vi "Fan Acceleration Curve J&J.vi"() -> ()   [LabVIEW 2015]
uses:
  <vilib>/Platform/TimedLoop/XDataNode/timing_clust.ctl
  <vilib>/Platform/TimedLoop/XDataNode/nitl_modes.ctl
  <vilib>/Platform/TimedLoop/XDataNode/wakeup.ctl
  <vilib>/platform/TimedLoop/XDataNode/XDataNode.xnode
  <vilib>/Platform/TimedLoop/XDataNode/XDNodeRunTimeDep.lvlib
panel:
  out "Countrate":cluster{i32[], i32[]}(graph)
  in  "Controls":T1
  in  "stop":bool
  out "counts per Time Increment":dbl(knob) scale=0.0..100.0
  out "output cluster":cluster{i32, dbl}
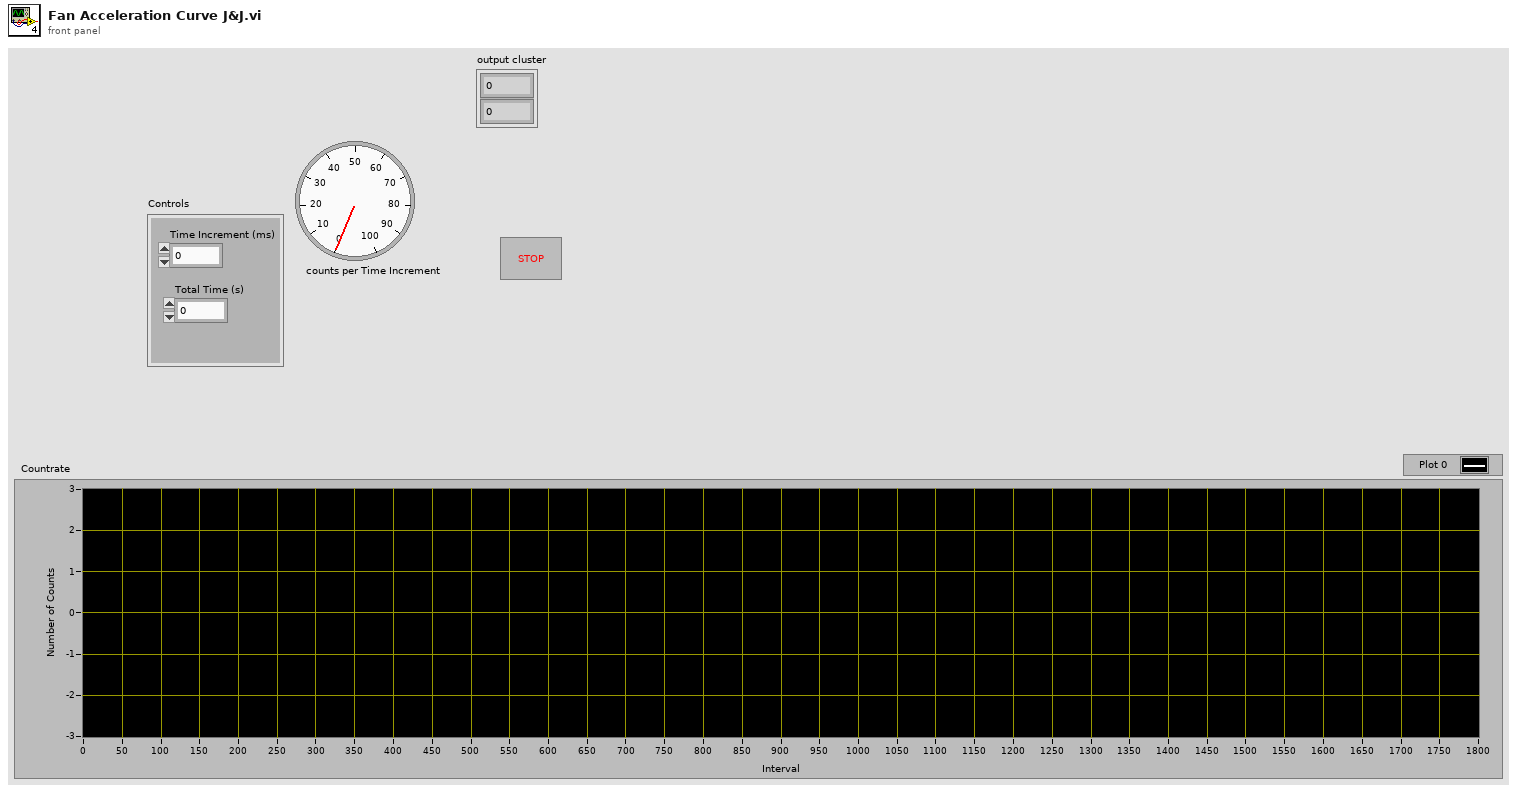
[diagram p1: front panel]
types:
  T1 = cluster{"Time Increment (ms)":i64, "Total Time (s)":dbl}
  T2 = enum16{"open", "replace", "create", "open or create", "replace or create", "replace or create with confirmation"}
  T3 = typedef "XDNodeRunTimeDep.lvlib/timing_clust.ctl" = cluster{"Expected End [f-1]":u64, "Actual End [f-1]":u64, "Finished Late? [f-1]":bool, "Expected End [i-1]":u64, "Actual End [i-1]":u64, "Finished Late? [i-1]":bool, "Expected Start [i]":u64, "Actual Start [i]":u64, "Expected Start [f]":u64, "Actual Start [f]":u64, "Source Name":string, "Structure Name":string, "Period":i64, "Deadline":i64, "Offset":i64, "Start":i64, "Priority":i32, "Timeout":i32, "Mode":T4, "Wakeup Reason":T5, "Error":errorcluster, "Source Type":string, "Secondary Source Type":string, "Global End Time":u64, "Global Start Time":u64, "Frame Duration":u64, "Iteration Duration":u64, "Assigned CPU":i32, "I/O Scan Engine Mode":u32}
  T4 = typedef "XDNodeRunTimeDep.lvlib/nitl_modes.ctl" = enum32{"No Change", "Process missed periods, maintain original phase", "Discard missed periods, maintain original phase", "Process missed periods, ignore original phase", "Discard missed periods, ignore original phase"}
  T5 = typedef "XDNodeRunTimeDep.lvlib/wakeup.ctl" = enum32{"Normal", "Aborted", "Asynchronous wakeup", "Timing source error", "Timed loop error", "Timeout"}
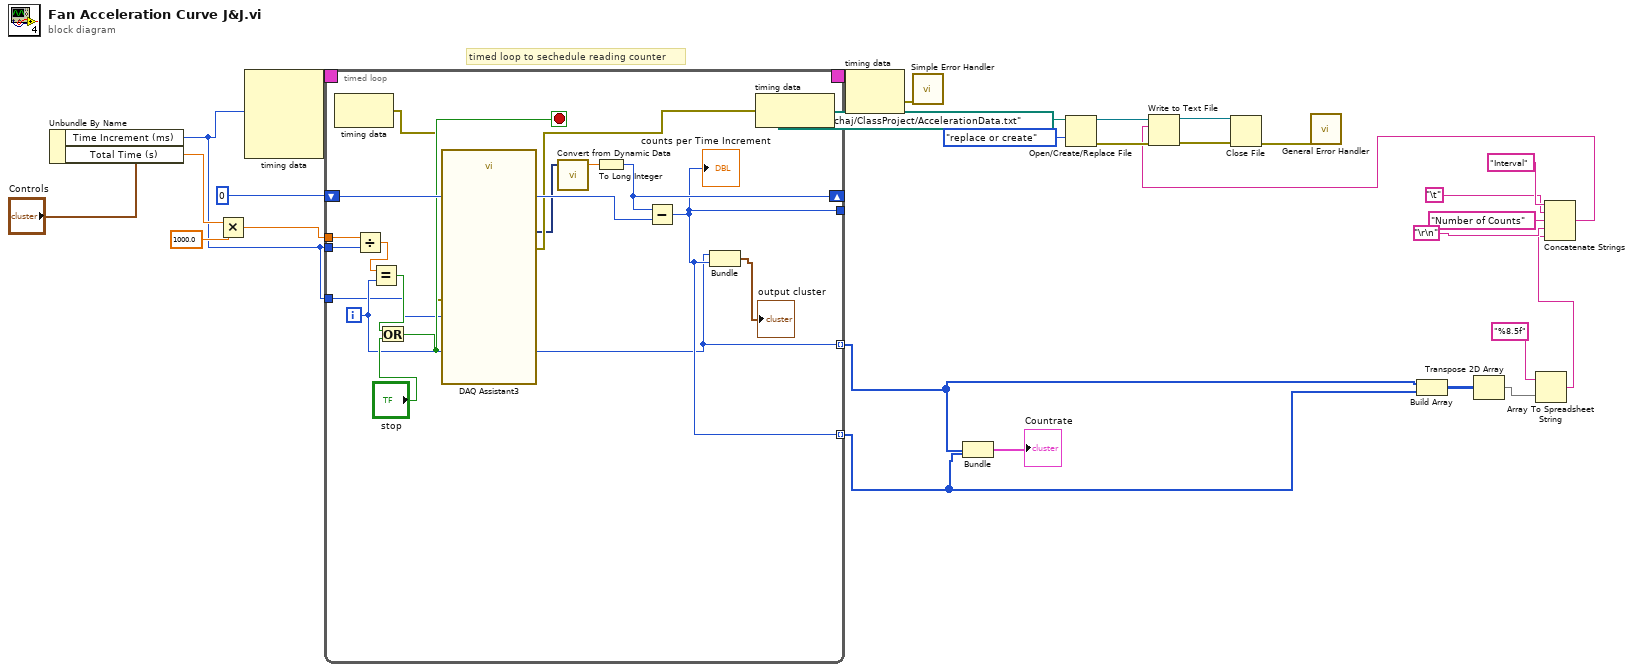
[diagram p0: block diagram]
diagram:
  # "timed loop to sechedule reading counter"
  n1 = Unbundle By Name("Controls") -> ("Time Increment (ms)"=w1:i64, "Total Time (s)"=w23:dbl)
  n2 = Multiply(x=w23, y=1000.0) -> (x*y=w21:dbl)
  n3 = node-c288(w1) -> (w28:T3)  [unwired: 3 in]
  n4 = timed-loop {
    timing: w28 -> [_]
    timing-out: [_] -> w27
    shift-right: [w44] -> _
    shift-left: 0 -> [w36]
    tunnel: [w38] -> _
    tunnel: w1 -> [w30]
    tunnel: w21 -> [w42]
    tunnel: [w38] -> w2 mode=indexing
    tunnel: [w37] -> w3 mode=indexing
    tunnel: w1 -> [w29]
    i -> [w37]
    stop <- w35 stop-if-true
    n5 = node-c288() -> (w33:errorcluster)  [unwired: 1 in]
    n6 = Divide(x=w42, y=w30) -> (x/y=w34:dbl)
    n7 = Equal?(x=w34, y=w37) -> (x = y?=w40:bool)
    n8 = Or(x=w40, y="stop") -> (x .or. y?=w35:bool)
    n9 = call "DAQ Assistant3"("number of samples"=w29, "error in"=w33, "stop (T)"=w35) -> ("data"=w31:dynamicdata, "error out"=w32:errorcluster)  [unwired: 14 in, 1 out]
    n10 = call "Convert from Dynamic Data"("Dynamic Data Type"=w31) -> ("Scalar"=w43:dbl)  [unwired: 3 in]
    n11 = To Long Integer(number=w43) -> (32bit integer=w44:i32)
    n12 = Subtract(x=w44, y=w36) -> (x-y=w38:i32)
    "counts per Time Increment" <- w38
    n13 = Bundle(w37, w38) -> (→"output cluster":cluster{i32, i32})  [unwired: 1 in]
    n14 = node-c288(w32) -> ()  [unwired: 1 out]
  }
  n15 = node-c288(w27) -> (w25:errorcluster)
  n16 = call <vilib>:"Simple Error Handler.vi"("error in (no error)"=w25) -> ()  [unwired: 4 in, 5 out]
  n17 = Bundle(w3, w2) -> (→"Countrate":cluster{i32[], i32[]})  [unwired: 1 in]
  n18 = Open/Create/Replace File(file path (use dialog)=path "C:/Users/atchaj/ClassProject/AccelerationData.txt", operation (0:open)=T2."replace or create") -> (refnum out=w16:refnum<file>, error out=w17:errorcluster)  [unwired: 4 in, 1 out]
  n19 = Build Array(w3, w2) -> (w4:i32[][])
  n20 = Transpose 2D Array(2D array=w4) -> (transposed array=w12:i32[][])
  n21 = Array To Spreadsheet String(array=w12, 3:"%8.5f" ("format string")) -> (spreadsheet string=w7:string)  [unwired: 1 in]
  n22 = Concatenate Strings("Interval" ("string"), "\t", "Number of Counts" ("string"), "\r\n", w7) -> (w6:string)
  n23 = Write to Text File(file (use dialog)=w16, text=w6, error in=w17) -> (refnum out=w15:refnum<file>, error out=w18:errorcluster)  [unwired: 1 in, 1 out]
  n24 = Close File(refnum=w15, error in=w18) -> (error out=w19:errorcluster)  [unwired: 1 out]
  n25 = call <vilib>:"General Error Handler.vi"("error in (no error)"=w19) -> ()  [unwired: 10 in, 5 out]
